vi "Build Modules.vi"(8 "error in (no error)":errorcluster, 11 "Item Ref in":T1 format="%.0x") -> (0 "error out":errorcluster, 2 "Modules":refnum<k24>[](array[refnum]), 3 "Item Ref out":T1 format="%.0x")   [LabVIEW 2014, in "SLSC configuration System Explorer.lvlib"]
uses:
  SLSC configuration System Explorer.lvlib
  <vilib>/NI Veristand/Custom Device API/Custom Device Item Ref.ctl
  Shared/Constants.vi
  <vilib>/NI Veristand/Custom Device API/Get Item Property (U16).vi
  <vilib>/NI Veristand/Custom Device API/Get Item Property (String).vi
  <vilib>/NI Veristand/Custom Device API/Get Item Property (U32).vi
  <vilib>/NI Veristand/Custom Device API/Custom Device API.lvlib
  Shared/SLSC configuration Shared.lvlib
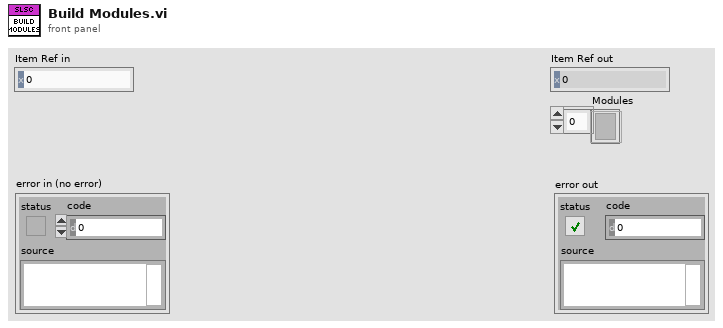
[diagram p1: front panel]
types:
  T1 = typedef "Custom Device API.lvlib/Custom Device Item Ref.ctl" = u64
  T2 = typedef "Custom Device API.lvlib/Custom Device Item Info.ctl" = cluster{"Name":string, "Is Channel":bool, "GUID":string, "Is Waveform":bool}
  T3 = typedef "SLSC configuration Shared.lvlib/Card Position.ctl" = cluster{"Rack #":u8, "Slot #":T4}
  T4 = typedef "SLSC configuration Shared.lvlib/Slot #.ctl" = u8
  T5 = typedef "Custom Device API.lvlib/Custom Device Channel.ctl" = cluster{"Type":T6, "Units":string, "Default Value":dbl, "Faultable":bool, "Scalable":bool}
  T6 = typedef "Custom Device API.lvlib/Custom Device Channel Type.ctl" = enum16{"Input", "Output"}
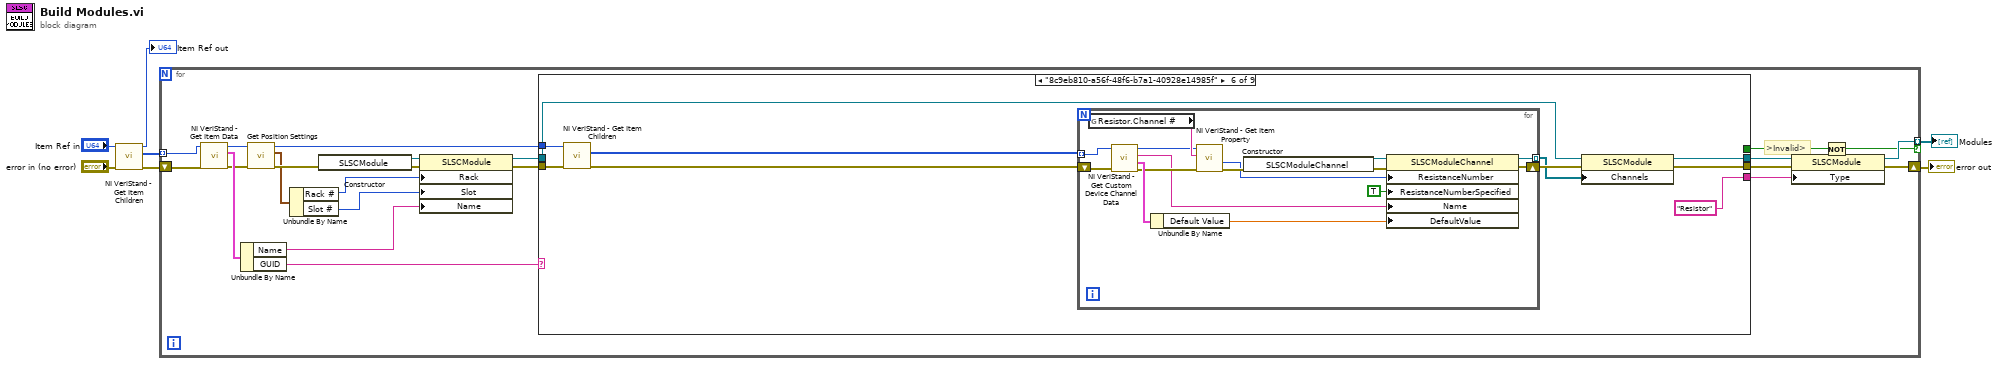
[diagram p0: block diagram]
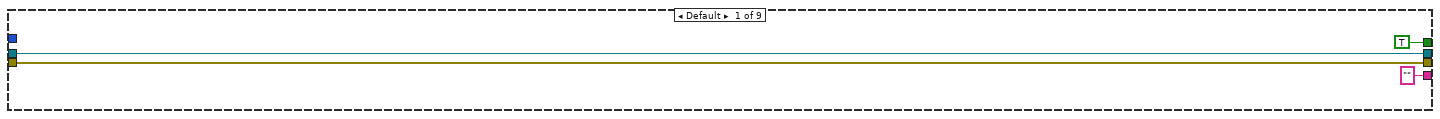
[diagram p2: hidden frame]
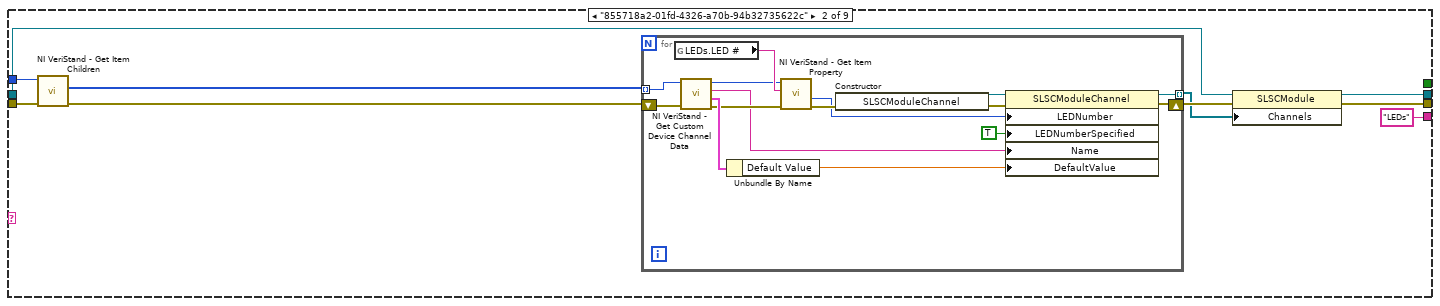
[diagram p3: hidden frame]
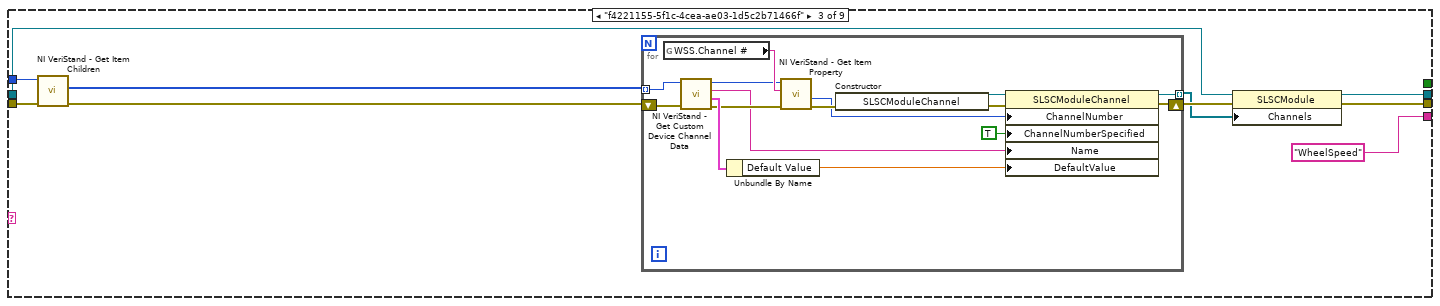
[diagram p4: hidden frame]
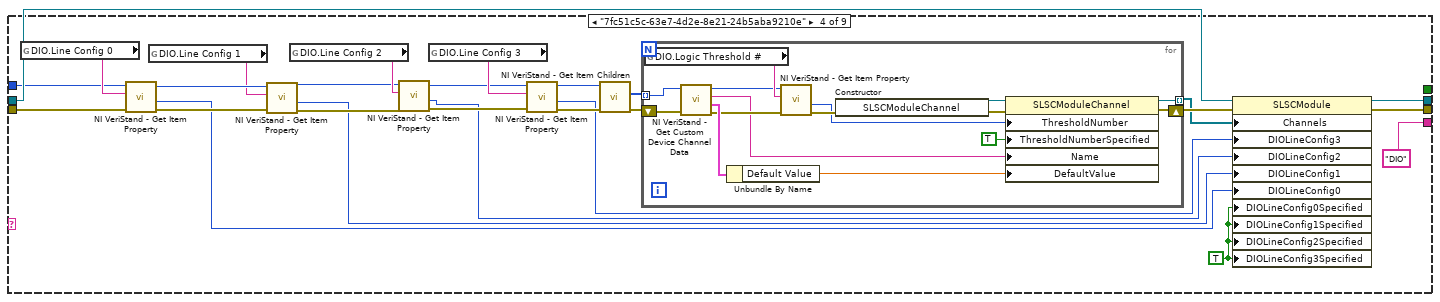
[diagram p5: hidden frame]
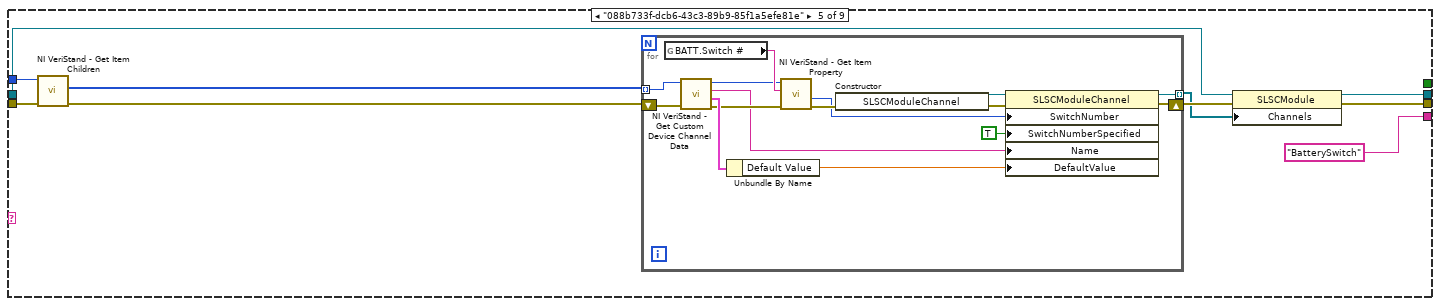
[diagram p6: hidden frame]
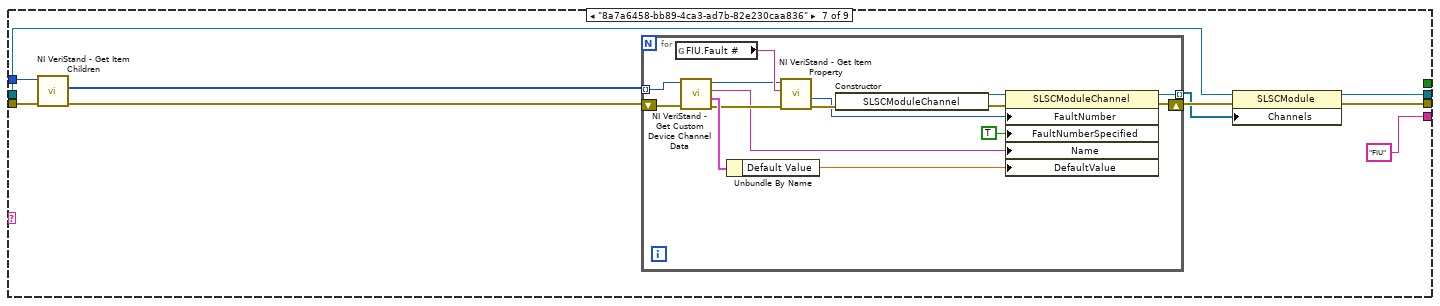
[diagram p7: hidden frame]
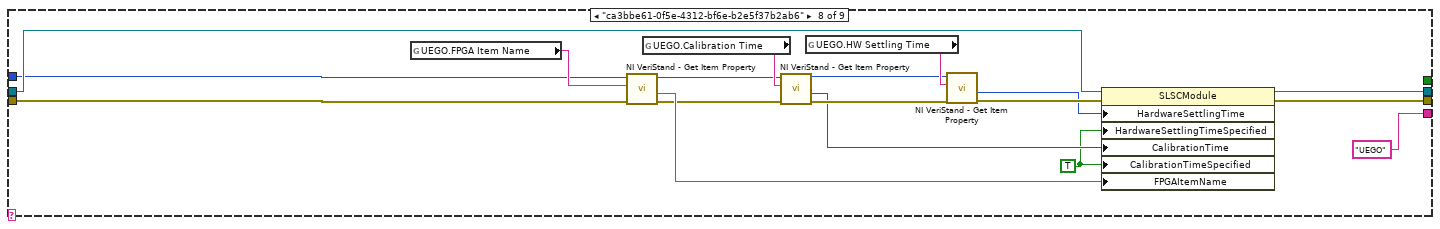
[diagram p8: hidden frame]
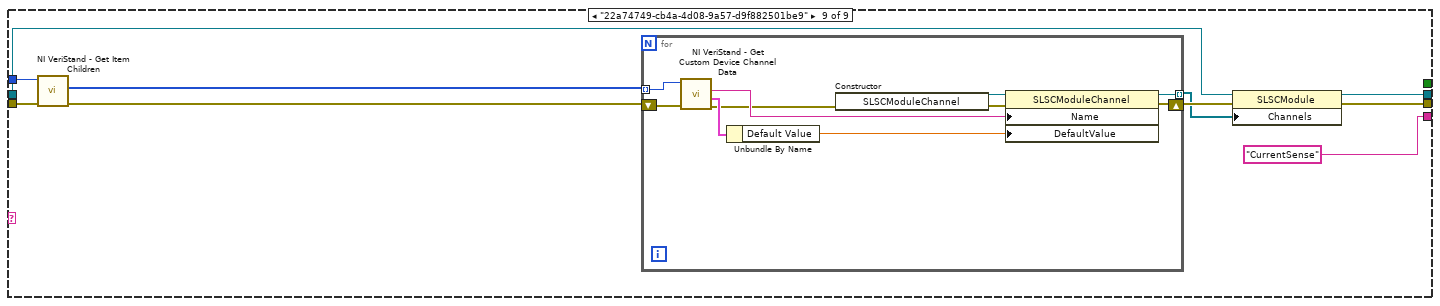
[diagram p9: hidden frame]
diagram:
  n1 = call <vilib>:"NI VeriStand - Get Item Children.vi"("error in (no error)"="error in (no error)", "Item Ref in"="Item Ref in") -> ("error out"=w5:errorcluster, "Child Refs"=w4:T1[], "Item Ref out"=→"Item Ref out":T1)  [unwired: 6 in, 1 out]
  n2 = for {
    tunnel: w4 -> [w29] mode=indexing
    shift-right: [w11] -> w1
    shift-left: w5 -> [w30]
    tunnel: [w10] -> w2 mode=indexing if=w8
    # ">Invalid>"
    n3 = call <vilib>:"NI VeriStand - Get Item Data.vi"("error in (no error)"=w30, "Item Ref in"=w29) -> ("error out"=w25:errorcluster, "Item Info"=w26:T2, "Item Ref out"=w24:T1)  [unwired: 6 in, 1 out]
    n4 = Unbundle By Name(w26) -> ("Name"=w22:string, "GUID"=w18:string)
    n5 = call "Get Position Settings.vi"("error in (no error)"=w25, "Item Ref in"=w24) -> ("error out"=w23:errorcluster, "Card Position"=w21:T3, "Item Ref out"=w12:T1)  [unwired: 7 in]
    n6 = Unbundle By Name(w21) -> ("Rack #"=w20:u8, "Slot #"=w19:T4)
    n7 = constructor class="SLSCModule"(error in=w23) -> (reference out=w28:refnum<k24>, error out=w27:errorcluster)  [unwired: 2 in, 1 out]
    n8 = property class="SLSCModule"(reference=w28, error in=w27, "Rack"=w20, "Slot"=w19, "Name"=w22) -> (reference out=w16:refnum<k24>, error out=w17:errorcluster)
    n9 = case shown="\"8c9eb810-a56f-48f6-b7a1-40928e14985f\"" w18 {
      tunnel: w17 -> [w34 w43 w68 w102 w135 w160 w185 w205 w228]
      tunnel: w16 -> [w33 w37 w62 w106 w129 w154 w179 w217 w222]
      tunnel: [w34 w38 w63 w107 w130 w155 w180 w218 w223] -> w15
      tunnel: [w33 w36 w61 w105 w128 w153 w178 w216 w221] -> w14
      tunnel: ["" ("Type") "LEDs" ("Type") "WheelSpeed" ("Type") "DIO" ("Type") "BatterySwitch" ("Type") "Resistor" ("Type") "FIU" ("Type") "UEGO" ("Type") "CurrentSense" ("Type")] -> w13
      tunnel: w12 -> [_ w42 w67 w101 w134 w159 w184 w203 w227]
      tunnel: [TRUE _ _ _ _ _ _ _ _] -> w9
      frame Default {
      }
      frame "855718a2-01fd-4326-a70b-94b32735622c" {
        n10 = call <vilib>:"NI VeriStand - Get Item Children.vi"("error in (no error)"=w43, "Item Ref in"=w42) -> ("error out"=w41:errorcluster, "Child Refs"=w40:T1[])  [unwired: 6 in, 2 out]
        n11 = for {
          shift-right: [w50] -> w39
          shift-left: w41 -> [w58]
          tunnel: w40 -> [w59] mode=indexing
          tunnel: [w45] -> w35 mode=indexing
          n12 = global read "Constants.vi" "LEDs.LED #"() -> (w56:string)
          n13 = call <vilib>:"NI VeriStand - Get Custom Device Channel Data.vi"("error in (no error)"=w58, "Channel Ref in"=w59) -> ("error out"=w55:errorcluster, "Channel"=w57:T5, "Channel Name"=w47:string, "Channel Ref out"=w54:T1)  [unwired: 4 in, 2 out]
          n14 = Unbundle By Name(w57) -> ("Default Value"=w46:dbl)
          n15 = call-poly <vilib>:"NI VeriStand - Get Item Property.vi"("error in (no error)"=w55, "Property Name"=w56, "Item Ref in"=w54) -> ("error out"=w53:errorcluster, "Value"=w49:u16)  [unwired: 5 in, 2 out]
          n16 = constructor class="SLSCModuleChannel"(error in=w53) -> (reference out=w51:refnum<k24>, error out=w52:errorcluster)  [unwired: 2 in, 1 out]
          n17 = property class="SLSCModuleChannel"(reference=w51, error in=w52, "LEDNumber"=w49, "LEDNumberSpecified"=TRUE, "Name"=w47, "DefaultValue"=w46) -> (reference out=w45:refnum<k24>, error out=w50:errorcluster)
        }
        n18 = property class="SLSCModule"(reference=w37, error in=w39, "Channels"=w35) -> (reference out=w36:refnum<k24>, error out=w38:errorcluster)
      }
      frame "f4221155-5f1c-4cea-ae03-1d5c2b71466f" {
        n19 = call <vilib>:"NI VeriStand - Get Item Children.vi"("error in (no error)"=w68, "Item Ref in"=w67) -> ("error out"=w66:errorcluster, "Child Refs"=w65:T1[])  [unwired: 6 in, 2 out]
        n20 = for {
          shift-right: [w75] -> w64
          shift-left: w66 -> [w83]
          tunnel: w65 -> [w84] mode=indexing
          tunnel: [w70] -> w60 mode=indexing
          n21 = global read "Constants.vi" "WSS.Channel #"() -> (w81:string)
          n22 = call <vilib>:"NI VeriStand - Get Custom Device Channel Data.vi"("error in (no error)"=w83, "Channel Ref in"=w84) -> ("error out"=w80:errorcluster, "Channel"=w82:T5, "Channel Name"=w72:string, "Channel Ref out"=w79:T1)  [unwired: 4 in, 2 out]
          n23 = Unbundle By Name(w82) -> ("Default Value"=w71:dbl)
          n24 = call-poly <vilib>:"NI VeriStand - Get Item Property.vi"("error in (no error)"=w80, "Property Name"=w81, "Item Ref in"=w79) -> ("error out"=w78:errorcluster, "Value"=w74:u16)  [unwired: 5 in, 2 out]
          n25 = constructor class="SLSCModuleChannel"(error in=w78) -> (reference out=w76:refnum<k24>, error out=w77:errorcluster)  [unwired: 2 in, 1 out]
          n26 = property class="SLSCModuleChannel"(reference=w76, error in=w77, "ChannelNumber"=w74, "ChannelNumberSpecified"=TRUE ("LEDNumberSpecified"), "Name"=w72, "DefaultValue"=w71) -> (reference out=w70:refnum<k24>, error out=w75:errorcluster)
        }
        n27 = property class="SLSCModule"(reference=w62, error in=w64, "Channels"=w60) -> (reference out=w61:refnum<k24>, error out=w63:errorcluster)
      }
      frame "7fc51c5c-63e7-4d2e-8e21-24b5aba9210e" {
        w85 = TRUE ("DIOLineConfig3Specified")
        n28 = global read "Constants.vi" "DIO.Line Config 0"() -> (w103:string)
        n29 = call-poly <vilib>:"NI VeriStand - Get Item Property.vi"("error in (no error)"=w102, "Property Name"=w103, "Item Ref in"=w101) -> ("error out"=w94:errorcluster, "Value"=w86:u16, "Item Ref out"=w93:T1)  [unwired: 5 in, 1 out]
        n30 = global read "Constants.vi" "DIO.Line Config 1"() -> (w90:string)
        n31 = call-poly <vilib>:"NI VeriStand - Get Item Property.vi"("error in (no error)"=w94, "Property Name"=w90, "Item Ref in"=w93) -> ("error out"=w92:errorcluster, "Value"=w87:u16, "Item Ref out"=w91:T1)  [unwired: 5 in, 1 out]
        n32 = global read "Constants.vi" "DIO.Line Config 2"() -> (w100:string)
        n33 = call-poly <vilib>:"NI VeriStand - Get Item Property.vi"("error in (no error)"=w92, "Property Name"=w100, "Item Ref in"=w91) -> ("error out"=w96:errorcluster, "Value"=w88:u16, "Item Ref out"=w95:T1)  [unwired: 5 in, 1 out]
        n34 = global read "Constants.vi" "DIO.Line Config 3"() -> (w97:string)
        n35 = call-poly <vilib>:"NI VeriStand - Get Item Property.vi"("error in (no error)"=w96, "Property Name"=w97, "Item Ref in"=w95) -> ("error out"=w99:errorcluster, "Value"=w89:u16, "Item Ref out"=w98:T1)  [unwired: 5 in, 1 out]
        n36 = call <vilib>:"NI VeriStand - Get Item Children.vi"("error in (no error)"=w99, "Item Ref in"=w98) -> ("error out"=w110:errorcluster, "Child Refs"=w109:T1[])  [unwired: 6 in, 2 out]
        n37 = for {
          shift-right: [w117] -> w108
          shift-left: w110 -> [w125]
          tunnel: w109 -> [w126] mode=indexing
          tunnel: [w112] -> w104 mode=indexing
          n38 = global read "Constants.vi" "DIO.Logic Threshold #"() -> (w123:string)
          n39 = call <vilib>:"NI VeriStand - Get Custom Device Channel Data.vi"("error in (no error)"=w125, "Channel Ref in"=w126) -> ("error out"=w122:errorcluster, "Channel"=w124:T5, "Channel Name"=w114:string, "Channel Ref out"=w121:T1)  [unwired: 4 in, 2 out]
          n40 = Unbundle By Name(w124) -> ("Default Value"=w113:dbl)
          n41 = call-poly <vilib>:"NI VeriStand - Get Item Property.vi"("error in (no error)"=w122, "Property Name"=w123, "Item Ref in"=w121) -> ("error out"=w120:errorcluster, "Value"=w116:u16)  [unwired: 5 in, 2 out]
          n42 = constructor class="SLSCModuleChannel"(error in=w120) -> (reference out=w118:refnum<k24>, error out=w119:errorcluster)  [unwired: 2 in, 1 out]
          n43 = property class="SLSCModuleChannel"(reference=w118, error in=w119, "ThresholdNumber"=w116, "ThresholdNumberSpecified"=TRUE ("LEDNumberSpecified"), "Name"=w114, "DefaultValue"=w113) -> (reference out=w112:refnum<k24>, error out=w117:errorcluster)
        }
        n44 = property class="SLSCModule"(reference=w106, error in=w108, "Channels"=w104, "DIOLineConfig3"=w89, "DIOLineConfig2"=w88, "DIOLineConfig1"=w87, "DIOLineConfig0"=w86, "DIOLineConfig0Specified"=w85, "DIOLineConfig1Specified"=w85, "DIOLineConfig2Specified"=w85, "DIOLineConfig3Specified"=w85) -> (reference out=w105:refnum<k24>, error out=w107:errorcluster)
      }
      frame "088b733f-dcb6-43c3-89b9-85f1a5efe81e" {
        n45 = call <vilib>:"NI VeriStand - Get Item Children.vi"("error in (no error)"=w135, "Item Ref in"=w134) -> ("error out"=w133:errorcluster, "Child Refs"=w132:T1[])  [unwired: 6 in, 2 out]
        n46 = for {
          shift-right: [w142] -> w131
          shift-left: w133 -> [w150]
          tunnel: w132 -> [w151] mode=indexing
          tunnel: [w137] -> w127 mode=indexing
          n47 = global read "Constants.vi" "BATT.Switch #"() -> (w148:string)
          n48 = call <vilib>:"NI VeriStand - Get Custom Device Channel Data.vi"("error in (no error)"=w150, "Channel Ref in"=w151) -> ("error out"=w147:errorcluster, "Channel"=w149:T5, "Channel Name"=w139:string, "Channel Ref out"=w146:T1)  [unwired: 4 in, 2 out]
          n49 = Unbundle By Name(w149) -> ("Default Value"=w138:dbl)
          n50 = call-poly <vilib>:"NI VeriStand - Get Item Property.vi"("error in (no error)"=w147, "Property Name"=w148, "Item Ref in"=w146) -> ("error out"=w145:errorcluster, "Value"=w141:u16)  [unwired: 5 in, 2 out]
          n51 = constructor class="SLSCModuleChannel"(error in=w145) -> (reference out=w143:refnum<k24>, error out=w144:errorcluster)  [unwired: 2 in, 1 out]
          n52 = property class="SLSCModuleChannel"(reference=w143, error in=w144, "SwitchNumber"=w141, "SwitchNumberSpecified"=TRUE ("LEDNumberSpecified"), "Name"=w139, "DefaultValue"=w138) -> (reference out=w137:refnum<k24>, error out=w142:errorcluster)
        }
        n53 = property class="SLSCModule"(reference=w129, error in=w131, "Channels"=w127) -> (reference out=w128:refnum<k24>, error out=w130:errorcluster)
      }
      frame "8c9eb810-a56f-48f6-b7a1-40928e14985f" {
        n54 = call <vilib>:"NI VeriStand - Get Item Children.vi"("error in (no error)"=w160, "Item Ref in"=w159) -> ("error out"=w158:errorcluster, "Child Refs"=w157:T1[])  [unwired: 6 in, 2 out]
        n55 = for {
          shift-right: [w167] -> w156
          shift-left: w158 -> [w175]
          tunnel: w157 -> [w176] mode=indexing
          tunnel: [w163] -> w152 mode=indexing
          n56 = global read "Constants.vi" "Resistor.Channel #"() -> (w173:string)
          n57 = call <vilib>:"NI VeriStand - Get Custom Device Channel Data.vi"("error in (no error)"=w175, "Channel Ref in"=w176) -> ("error out"=w172:errorcluster, "Channel"=w174:T5, "Channel Name"=w164:string, "Channel Ref out"=w171:T1)  [unwired: 4 in, 2 out]
          n58 = Unbundle By Name(w174) -> ("Default Value"=w162:dbl)
          n59 = call-poly <vilib>:"NI VeriStand - Get Item Property.vi"("error in (no error)"=w172, "Property Name"=w173, "Item Ref in"=w171) -> ("error out"=w170:errorcluster, "Value"=w166:u16)  [unwired: 5 in, 2 out]
          n60 = constructor class="SLSCModuleChannel"(error in=w170) -> (reference out=w168:refnum<k24>, error out=w169:errorcluster)  [unwired: 2 in, 1 out]
          n61 = property class="SLSCModuleChannel"(reference=w168, error in=w169, "ResistanceNumber"=w166, "ResistanceNumberSpecified"=TRUE ("LEDNumberSpecified"), "Name"=w164, "DefaultValue"=w162) -> (reference out=w163:refnum<k24>, error out=w167:errorcluster)
        }
        n62 = property class="SLSCModule"(reference=w154, error in=w156, "Channels"=w152) -> (reference out=w153:refnum<k24>, error out=w155:errorcluster)
      }
      frame "8a7a6458-bb89-4ca3-ad7b-82e230caa836" {
        n63 = call <vilib>:"NI VeriStand - Get Item Children.vi"("error in (no error)"=w185, "Item Ref in"=w184) -> ("error out"=w183:errorcluster, "Child Refs"=w182:T1[])  [unwired: 6 in, 2 out]
        n64 = for {
          shift-right: [w192] -> w181
          shift-left: w183 -> [w200]
          tunnel: w182 -> [w201] mode=indexing
          tunnel: [w187] -> w177 mode=indexing
          n65 = global read "Constants.vi" "FIU.Fault #"() -> (w198:string)
          n66 = call <vilib>:"NI VeriStand - Get Custom Device Channel Data.vi"("error in (no error)"=w200, "Channel Ref in"=w201) -> ("error out"=w197:errorcluster, "Channel"=w199:T5, "Channel Name"=w189:string, "Channel Ref out"=w196:T1)  [unwired: 4 in, 2 out]
          n67 = Unbundle By Name(w199) -> ("Default Value"=w188:dbl)
          n68 = call-poly <vilib>:"NI VeriStand - Get Item Property.vi"("error in (no error)"=w197, "Property Name"=w198, "Item Ref in"=w196) -> ("error out"=w195:errorcluster, "Value"=w191:u16)  [unwired: 5 in, 2 out]
          n69 = constructor class="SLSCModuleChannel"(error in=w195) -> (reference out=w193:refnum<k24>, error out=w194:errorcluster)  [unwired: 2 in, 1 out]
          n70 = property class="SLSCModuleChannel"(reference=w193, error in=w194, "FaultNumber"=w191, "FaultNumberSpecified"=TRUE ("LEDNumberSpecified"), "Name"=w189, "DefaultValue"=w188) -> (reference out=w187:refnum<k24>, error out=w192:errorcluster)
        }
        n71 = property class="SLSCModule"(reference=w179, error in=w181, "Channels"=w177) -> (reference out=w178:refnum<k24>, error out=w180:errorcluster)
      }
      frame "ca3bbe61-0f5e-4312-bf6e-b2e5f37b2ab6" {
        w208 = TRUE ("CalibrationTimeSpecified")
        n72 = global read "Constants.vi" "UEGO.FPGA Item Name"() -> (w204:string)
        n73 = call-poly <vilib>:"NI VeriStand - Get Item Property.vi"("error in (no error)"=w205, "Property Name"=w204, "Item Ref in"=w203) -> ("error out"=w206:errorcluster, "Value"=w207:string, "Item Ref out"=w202:T1)  [unwired: 5 in, 1 out]
        n74 = global read "Constants.vi" "UEGO.Calibration Time"() -> (w215:string)
        n75 = call-poly <vilib>:"NI VeriStand - Get Item Property.vi"("error in (no error)"=w206, "Property Name"=w215, "Item Ref in"=w202) -> ("error out"=w213:errorcluster, "Value"=w209:u32, "Item Ref out"=w212:T1)  [unwired: 5 in, 1 out]
        n76 = global read "Constants.vi" "UEGO.HW Settling Time"() -> (w214:string)
        n77 = call-poly <vilib>:"NI VeriStand - Get Item Property.vi"("error in (no error)"=w213, "Property Name"=w214, "Item Ref in"=w212) -> ("error out"=w211:errorcluster, "Value"=w210:u32)  [unwired: 5 in, 2 out]
        n78 = property class="SLSCModule"(reference=w217, error in=w211, "HardwareSettlingTime"=w210, "HardwareSettlingTimeSpecified"=w208, "CalibrationTime"=w209, "CalibrationTimeSpecified"=w208, "FPGAItemName"=w207) -> (reference out=w216:refnum<k24>, error out=w218:errorcluster)
      }
      frame "22a74749-cb4a-4d08-9a57-d9f882501be9" {
        n79 = call <vilib>:"NI VeriStand - Get Item Children.vi"("error in (no error)"=w228, "Item Ref in"=w227) -> ("error out"=w226:errorcluster, "Child Refs"=w225:T1[])  [unwired: 6 in, 2 out]
        n80 = for {
          shift-right: [w234] -> w224
          shift-left: w226 -> [w238]
          tunnel: w225 -> [w239] mode=indexing
          tunnel: [w231] -> w220 mode=indexing
          n81 = call <vilib>:"NI VeriStand - Get Custom Device Channel Data.vi"("error in (no error)"=w238, "Channel Ref in"=w239) -> ("error out"=w230:errorcluster, "Channel"=w237:T5, "Channel Name"=w233:string)  [unwired: 4 in, 3 out]
          n82 = Unbundle By Name(w237) -> ("Default Value"=w232:dbl)
          n83 = constructor class="SLSCModuleChannel"(error in=w230) -> (reference out=w235:refnum<k24>, error out=w236:errorcluster)  [unwired: 2 in, 1 out]
          n84 = property class="SLSCModuleChannel"(reference=w235, error in=w236, "Name"=w233, "DefaultValue"=w232) -> (reference out=w231:refnum<k24>, error out=w234:errorcluster)
        }
        n85 = property class="SLSCModule"(reference=w222, error in=w224, "Channels"=w220) -> (reference out=w221:refnum<k24>, error out=w223:errorcluster)
      }
    }
    n86 = property class="SLSCModule"(reference=w14, error in=w15, "Type"=w13) -> (reference out=w10:refnum<k24>, error out=w11:errorcluster)
    n87 = Not(x=w9) -> (.not. x?=w8:bool)
  }
  "Modules" <- w2
  "error out" <- w1
